vi "setIntegerField.vi"(8 "error in (no error)":errorcluster, 9 "Value String":string, 10 "Field Name":string, 11 "PulseData in":refnum<class "PulseData.lvclass">) -> (0 "error out":errorcluster, 3 "PulseData out":refnum<class "PulseData.lvclass">)   [LabVIEW 2013, in "Controls Log Monitor.lvlib" / "PulseData.lvclass"]
uses:
  PulseData.lvclass
  PulseData.lvclass/PulseData.ctl
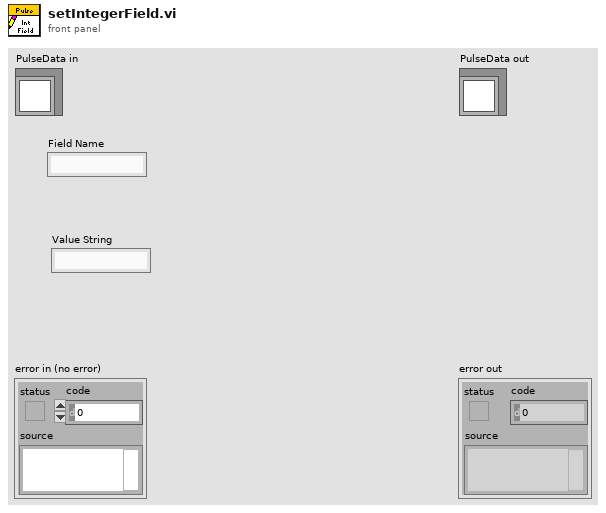
[diagram p1: front panel]
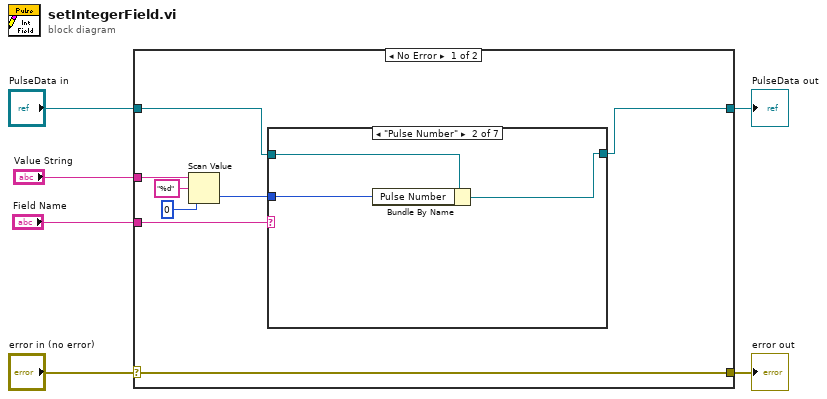
[diagram p0: block diagram]
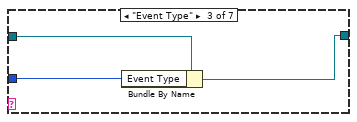
[diagram p3: hidden frame]
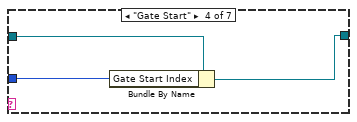
[diagram p4: hidden frame]
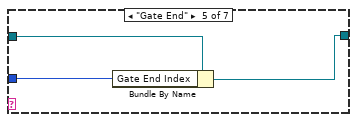
[diagram p5: hidden frame]
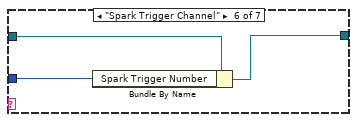
[diagram p6: hidden frame]
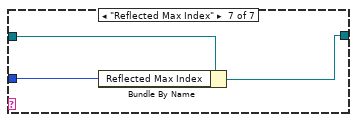
[diagram p7: hidden frame]
diagram:
  n1 = case shown="No Error" "error in (no error)" {
    selector: "error in (no error)" -> [w14 w35]
    tunnel: [w14 w35] -> w5
    tunnel: [w9 w34] -> w3
    tunnel: "PulseData in" -> [w13 w34]
    tunnel: "Field Name" -> [w12 _]
    tunnel: "Value String" -> [w8 _]
    frame No Error {
      n2 = Scan Value(string=w8, format string="%d", default (0 dbl)=0) -> (value=w10:i32)  [unwired: 1 out]
      n3 = case shown="\"Pulse Number\"" w12 {
        tunnel: w13 -> [w15 w18 w21 w24 w27 w30 w33]
        tunnel: w10 -> [_ w17 w20 w23 w26 w29 w32]
        tunnel: [w15 w16 w19 w22 w25 w28 w31] -> w9
        frame Default {
        }
        frame "Pulse Number" {
          n4 = Bundle By Name(cluster=w18, "Pulse Number"=w17) -> (w16:refnum<class "PulseData.lvclass">)
        }
        frame "Event Type" {
          n5 = Bundle By Name(cluster=w21, "Event Type"=w20) -> (w19:refnum<class "PulseData.lvclass">)
        }
        frame "Gate Start" {
          n6 = Bundle By Name(cluster=w24, "Gate Start Index"=w23) -> (w22:refnum<class "PulseData.lvclass">)
        }
        frame "Gate End" {
          n7 = Bundle By Name(cluster=w27, "Gate End Index"=w26) -> (w25:refnum<class "PulseData.lvclass">)
        }
        frame "Spark Trigger Channel" {
          n8 = Bundle By Name(cluster=w30, "Spark Trigger Number"=w29) -> (w28:refnum<class "PulseData.lvclass">)
        }
        frame "Reflected Max Index" {
          n9 = Bundle By Name(cluster=w33, "Reflected Max Index"=w32) -> (w31:refnum<class "PulseData.lvclass">)
        }
      }
    }
    frame Error {
    }
  }
  "error out" <- w5
  "PulseData out" <- w3
